vi "mod_FM CE Modulation v2.vi"(6 "reset?":bool, 7 "carrier phase [rad]":dbl format="%.2f", 8 "kf":dbl format="%.2f", 10 "fs":dbl format="%.2f", 11 "x":dbl[](array[numeric]) format="%.2f") -> (3 "FM CE":cdb[](array[numeric]) format="%.2f")   [LabVIEW 2020, in "niAMT.lvlib"]
doc: "This VI performs FM modulation of incoming message signal. The output of this VI is the base band complex envelope of FM modulated signal."
uses:
  <vilib>/addons/Modulation/niAMT.lvlib
  <vilib>/addons/Modulation/Analog/support/mod_Modulo Integrator (real array).vi
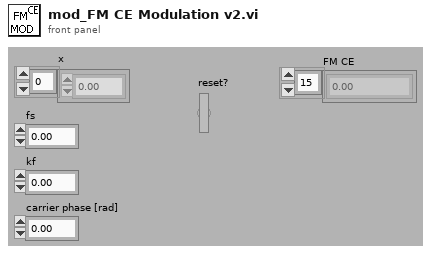
[diagram p1: front panel]
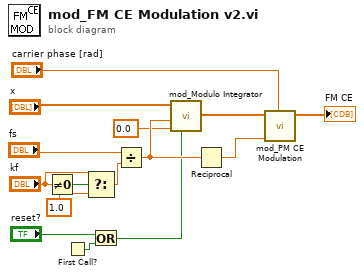
[diagram p0: block diagram]
diagram:
  n1 = Not Equal To 0?(x="kf") -> (x != 0?=w11:bool)
  n2 = First Call?() -> (First Call?: T/F=w1:bool)
  n3 = Select(t="kf", s=w11, f=1.0 ("lower limit")) -> (s? t:f=w6:dbl)
  n4 = Or(x="reset?", y=w1) -> (x .or. y?=w2:bool)
  n5 = Divide(x="fs", y=w6) -> (x/y=w4:dbl)
  n6 = call-poly <vilib>:"mod_Modulo Integrator.vi"("reset?"=w2, "initial y"=0.0, "modulo"=w4, "x"="x") -> ("y"=w12:dbl[])  [unwired: 7 out]
  n7 = Reciprocal(x=w4) -> (1/x=w5:dbl)
  n8 = call <vilib>:"mod_PM CE Modulation.vi"("carrier phase (rad)"="carrier phase [rad]", "kp"=w5, "x"=w12) -> ("PM CE"=→"FM CE":cdb[])  [unwired: 8 out]
